vi "Test UI.vi"() -> ()   [LabVIEW 2018]
panel:
  in  "Blank Button":bool
  in  "Stop Button":bool
  in  "OK Button 3":bool
  in  "OK Button 2":bool
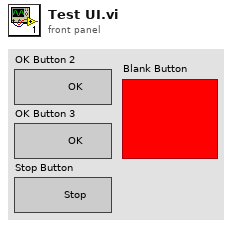
[diagram p1: front panel]
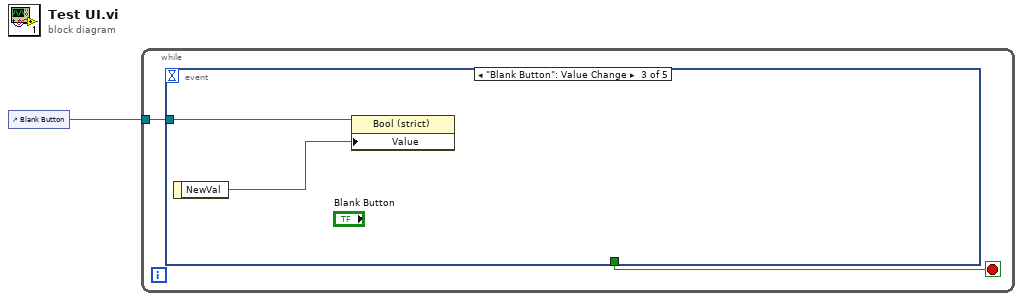
[diagram p0: block diagram]
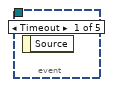
[diagram p2: hidden frame]
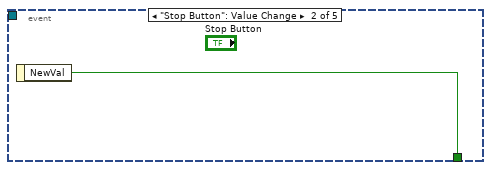
[diagram p3: hidden frame]
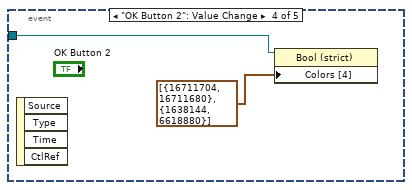
[diagram p4: hidden frame]
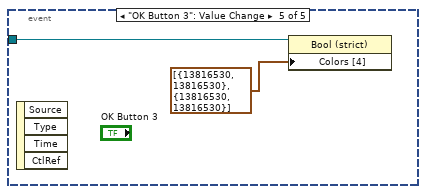
[diagram p5: hidden frame]
diagram:
  n1 = control-ref of="Blank Button"() -> (w1:refnum<vi>)
  n2 = while {
    tunnel: w1 -> [w2]
    stop <- w3 stop-if-true
    n3 = event shown="[2] \"Blank Button\": Value Change" {
      selector: _ -> [_ _ _ _ _]
      dyn-events: _ -> [_ _ _ _ _]
      timeout: _ -> [_ _ _ _ _]
      tunnel: [_ w4 _ _ _] -> w3
      tunnel: w2 -> [_ _ w6 w7 w9]
      event Timeout {
        n4 = event-data() -> ()  [unwired: 1 in, 1 out]
      }
      event "Stop Button": Value Change {
        n5 = event-data() -> ("NewVal"=w4:bool)  [unwired: 1 in]
      }
      event "Blank Button": Value Change {
        n6 = event-data() -> ("NewVal"=w5:bool)  [unwired: 1 in]
        n7 = property class="Bool (strict)"(reference=w6, "Value"=w5) -> ()  [unwired: 1 in, 2 out]
      }
      event "OK Button 2": Value Change {
        n8 = event-data() -> ()  [unwired: 1 in, 4 out]
        n9 = property class="Bool (strict)"(reference=w7, "Colors [4]"=cluster{u32, u32}[] [{16711704, 16711680}, {1638144, 6618880}]) -> ()  [unwired: 1 in, 2 out]
      }
      event "OK Button 3": Value Change {
        n10 = event-data() -> ()  [unwired: 1 in, 4 out]
        n11 = property class="Bool (strict)"(reference=w9, "Colors [4]"=cluster{u32, u32}[] [{13816530, 13816530}, {13816530, 13816530}]) -> ()  [unwired: 1 in, 2 out]
      }
    }
  }
